vi "niRFUtil CFG INI File Key.vi"(0 "File In":path, 5 "Section":string, 7 "Key Name":string, 9 "Write String":string, 11 "error in (no error)":errorcluster, 13 "Action (Read)":enum16{"Read", "Write", "Delete"}(ring)) -> (4 "dup File":path, 6 "Key Item":string, 15 "error out":errorcluster)   [LabVIEW 2015, in "niRFUtil.lvlib"]
doc: "The Modify INI File VI allows the user to read or write entries in a text file that is in the standard Windows INI file format. \n\nThe Read Action searches the specified initialization file for a key that matches the name specified by the Key Name control under the section heading specified by the Section control. If it finds the key, the function retrieves the corresponding string to the Returned String indicator. If the key does not exist, the function returns a null string. A section in the initialization file must have the following form: \n\n[section]\nkey=string\n .\n .\n .\n\nThe Write action adds or modifies entries to the INI file.\n\nThe Delete Action deletes entries in the specified section.\n\n(c) Copyright 2007, National Instruments, Inc. This software may not be duplicated, sold, or distributed without written consent from National Instruments."
uses:
  niRFUtil.lvlib
  kernel32.dll
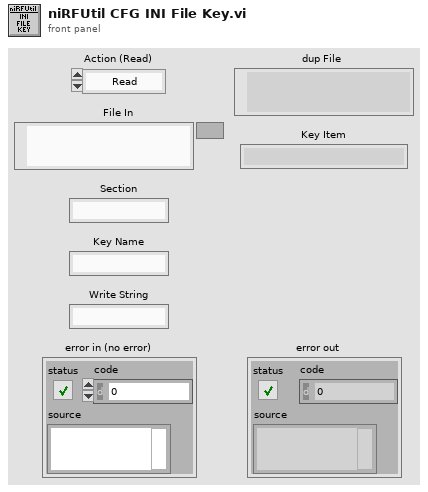
[diagram p1: front panel]
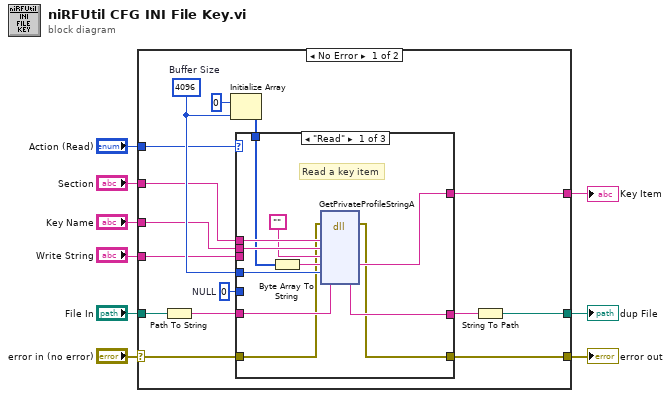
[diagram p0: block diagram]
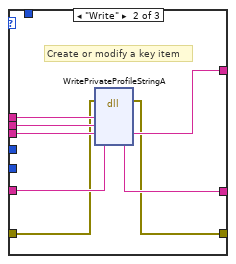
[diagram p2: hidden frame]
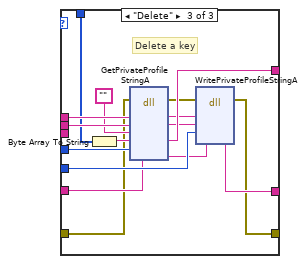
[diagram p3: hidden frame]
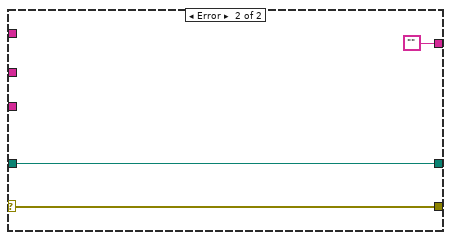
[diagram p4: hidden frame]
diagram:
  n1 = case shown="No Error" "error in (no error)" {
    selector: "error in (no error)" -> [w12 w61]
    tunnel: [w10 w61] -> w9
    tunnel: [w20 ""] -> w8
    tunnel: "Action (Read)" -> [w19 _]
    tunnel: "Section" -> [w13 _]
    tunnel: "Key Name" -> [w18 _]
    tunnel: "Write String" -> [w17 _]
    tunnel: "File In" -> [w16 w60]
    tunnel: [w11 w60] -> w1
    frame No Error {
      w21 = 0  # NULL
      w24 = 4096  # Buffer Size
      n2 = Path To String(path=w16) -> (string=w15:string)
      n3 = Initialize Array(u8 0, w24) -> (w23:u8[])
      n4 = case shown="\"Read\"" w19 {
        tunnel: w13 -> [w35 w43 w59]
        tunnel: w18 -> [w34 w41 w58]
        tunnel: w17 -> [_ w42 _]
        tunnel: w24 -> [w33 _ w57]
        tunnel: w23 -> [w32 _ w56]
        tunnel: w21 -> [_ _ w55]
        tunnel: [w31 w40 w54] -> w20
        tunnel: w15 -> [w29 w39 w48]
        tunnel: [w28 w38 w49] -> w14
        tunnel: w12 -> [w26 w37 w46]
        tunnel: [w25 w36 w44] -> w10
        frame "Read" {
          # "Read a key item"
          n5 = Byte Array To String(unsigned byte array=w32) -> (string=w30:string)
          n6 = dll-call lib="Kernel32.dll" fn="GetPrivateProfileStringA" label="Read"(error in=w26, "AppName"=w35, "KeyName"=w34, "Default"="", "ReturnedString"=w30, "Size"=w33, "FileName"=w29) -> (error out=w25:errorcluster, "ReturnedString"=w31:string, "FileName"=w28:string)  [unwired: 5 in, 3 out]
        }
        frame "Write" {
          # "Create or modify a key item"
          n7 = dll-call lib="Kernel32.dll" fn="WritePrivateProfileStringA" label="Write"(error in=w37, "AppName"=w43, "KeyName"=w41, "String"=w42, "FileName"=w39) -> (error out=w36:errorcluster, "String"=w40:string, "FileName"=w38:string)  [unwired: 4 in, 2 out]
        }
        frame "Delete" {
          # "Delete a key"
          n8 = Byte Array To String(unsigned byte array=w56) -> (string=w52:string)
          n9 = dll-call lib="Kernel32.dll" fn="GetPrivateProfileStringA" label="Read"(error in=w46, "AppName"=w59, "KeyName"=w58, "Default"="", "ReturnedString"=w52, "Size"=w57, "FileName"=w48) -> (error out=w45:errorcluster, "AppName"=w51:string, "KeyName"=w50:string, "ReturnedString"=w54:string, "FileName"=w53:string)  [unwired: 3 in, 3 out]
          n10 = dll-call lib="Kernel32.dll" fn="WritePrivateProfileStringA" label="Delete"(error in=w45, "AppName"=w51, "KeyName"=w50, "String"=w55, "FileName"=w53) -> (error out=w44:errorcluster, "FileName"=w49:string)  [unwired: 5 in, 2 out]
        }
      }
      n11 = String To Path(string=w14) -> (path=w11:path)
    }
    frame Error {
    }
  }
  "error out" <- w9
  "Key Item" <- w8
  "dup File" <- w1
